vi "Icon_Update Template icon array.vi"(8 "Error":errorcluster, 9 "Format":T1={"Color"={"Body txt"=255, "Body Back"=12632256, "Frame"=0, "Header txt"=32768, "Header Back"=16744703, "type"=enum."2 Color"}, "Icon Sizing"={"Rule"=enum."Static", "Header"=TRUE, "Rows"=5, "Width"=32, "Position"=enum."MID-CTR"}} {"Icon Sizing"."Rows" min=1 max=5 step=1; "Icon Sizing"."Width" min=7 max=32 step=1}, 10 "Header":T7, 11 "Template Array":T8[](array[typedef]) {"Format"."Icon Sizing"."Rows" min=1 max=5 step=1; "Format"."Icon Sizing"."Width" min=7 max=32 step=1}) -> (0 "Error Out":errorcluster, 3 "Template Array Out":T8[](array[typedef]) {"Format"."Icon Sizing"."Rows" min=1 max=5 step=1; "Format"."Icon Sizing"."Width" min=7 max=32 step=1})   [LabVIEW 2009]
doc: "Adds and Updates the Color Cluster array"
uses:
  Controls/Cluster/Cluster_Format Storage.ctl
  Controls/String_Picture/STRING_Line Display.ctl
  Controls/Cluster/Cluster_Icon Format.ctl
  Controls/Cluster/Cluster_Icon Color Set.ctl
  Controls/Enum/ENUM_Frame Template Select.ctl
  Controls/Cluster/Cluster_Sizing Data.ctl
  Controls/Enum/ENUM_Icon Sizing.ctl
  Controls/Enum/RBENUM_Icon Position.ctl
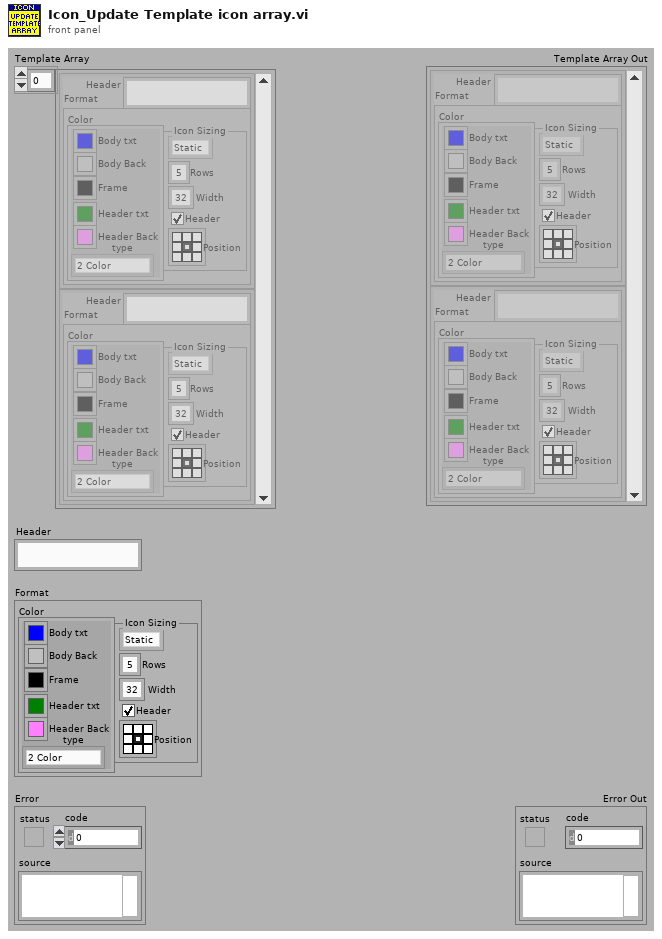
[diagram p1: front panel]
types:
  T1 = typedef "Cluster_Icon Format.ctl" = cluster{"Color":T2, "Icon Sizing":T4}
  T2 = typedef "Cluster_Icon Color Set.ctl" = cluster{"Body txt":u32, "Body Back":u32, "Frame":u32, "Header txt":u32, "Header Back":u32, "type":T3}
  T3 = typedef "ENUM_Frame Template Select.ctl" = enum16{"2 Color", "5 Color"}
  T4 = typedef "Cluster_Sizing Data.ctl" = cluster{"Rule":T5, "Header":bool, "Rows":u32, "Width":u32, "Position":T6}
  T5 = typedef "ENUM_Icon Sizing.ctl" = enum16{"Static", "Auto"}
  T6 = typedef "RBENUM_Icon Position.ctl" = enum32{"LFT-TOP", "MID-TOP", "RGT-TOP", "LFT-CTR", "MID-CTR", "RGT-CTR", "LFT-BOT", "MID-BOT", "RGT-BOT"}
  T7 = typedef "STRING_Line Display.ctl" = string
  T8 = typedef "Cluster_Format Storage.ctl" = cluster{"Header":T7, "Format":T1}
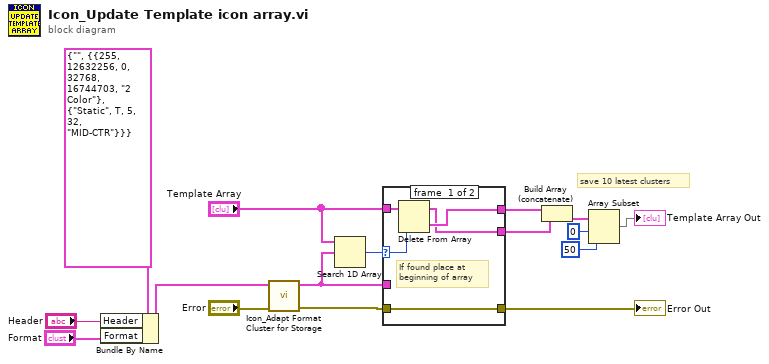
[diagram p0: block diagram]
diagram:
  # "save 10 latest clusters"
  n1 = Bundle By Name(cluster=T8 {"Header"="", "Format"={"Color"={"Body txt"=255, "Body Back"=12632256, "Frame"=0, "Header txt"=32768, "Header Back"=16744703, "type"=enum."2 Color"}, "Icon Sizing"={"Rule"=enum."Static", "Header"=TRUE, "Rows"=5, "Width"=32, "Position"=enum."MID-CTR"}}} ("Format Storage"), "Header"="Header", "Format"="Format") -> (w3:T8)
  n2 = call "Icon_Adapt Format Cluster for Storage.vi"("Error"="Error", "Colors"=w3) -> ("Error Out"=w7:errorcluster, "Colors Out"=w5:T8)  [unwired: 8 in]
  n3 = Search 1D Array(1D array="Template Array", element=w5) -> (index of element=w16:i32)  [unwired: 1 in]
  n4 = case shown="Default" w16 {
    selector: w16 -> [w19 _]
    tunnel: w5 -> [_ w23]
    tunnel: "Template Array" -> [w20 w22]
    tunnel: w7 -> [w21 w24]
    tunnel: [w21 w24] -> w10
    tunnel: [w18 w23] -> w13
    tunnel: [w17 w22] -> w9
    frame #0 {
      # "If found place at\nbeginning of array"
      n5 = Delete From Array(array=w20, index=w19) -> (deleted portion=w18:T8, array with subset deleted=w17:T8[])  [unwired: 1 in]
    }
    frame #1 {
      # "If not found place at\nbeginning of array."
    }
  }
  "Error Out" <- w10
  n6 = Build Array (concatenate)(w13, w9) -> (w14:T8[])
  n7 = Array Subset(array=w14, index=0, length=50) -> (→"Template Array Out":T8[])
